vi "getKeepAlive.vi"(11 "CONNECT in":refnum<class "CONNECT.lvclass">) -> (2 "Keep Alive (s)":u16, 3 "CONNECT out":refnum<class "CONNECT.lvclass">)   [LabVIEW 2013, in "MQTT_Control_Packets.lvlib" / "CONNECT.lvclass"]
uses:
  CONNECT.lvclass
  ControlPacket/ControlPacket.lvclass/ControlPacket.ctl
  ControlPacket/ControlPacket.lvclass
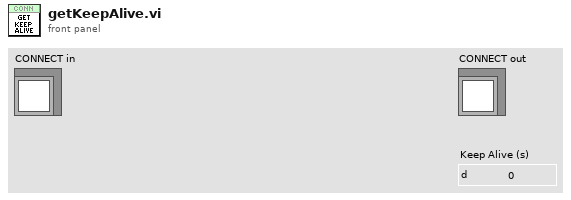
[diagram p1: front panel]
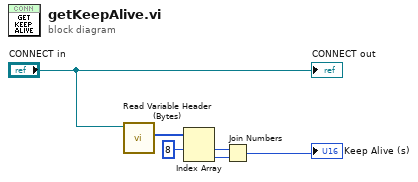
[diagram p0: block diagram]
diagram:
  n1 = call "Read Variable Header (Bytes).vi"("ControlPacket in"="CONNECT in") -> ("Variable Header (Bytes)"=w5:u8[])  [unwired: 9 in, 1 out]
  n2 = Index Array(array=w5, index #1=8 ("index")) -> (element #1=w4:u8, element #2=w3:u8)  [unwired: 1 in]
  n3 = Join Numbers(hi=w4, lo=w3) -> ((hi.lo)=→"Keep Alive (s)":u16)
  "CONNECT out" <- "CONNECT in"
